vi "getTagDataBytes.vi"(10 "Data Arry":u8[](array[numeric]) format="%x") -> (2 "Bytes":u8)   [LabVIEW 2018]
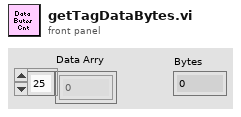
[diagram p1: front panel]
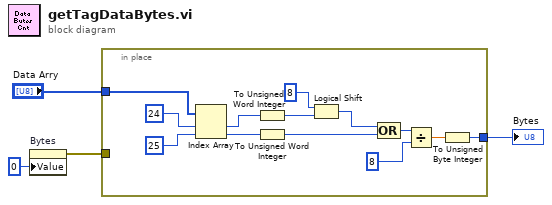
[diagram p0: block diagram]
diagram:
  n1 = property on="Bytes" class="DigNum (strict)"("Value"=u8 0 ("Butes")) -> (error out=w1:errorcluster)  [unwired: 2 in, 1 out]
  n2 = in-place {
    in-place-border: "Data Arry" -> [w17]
    in-place-border: [w5] -> w3
    in-place-border: w1 -> [_]
    n3 = Index Array(array=w17, index #1=24 ("index"), index #2=25 ("index")) -> (element #1=w14:u8, element #2=w13:u8)
    n4 = To Unsigned Word Integer(number=w14) -> (unsigned 16bit integer=w12:u16)
    n5 = To Unsigned Word Integer(number=w13) -> (unsigned 16bit integer=w9:u16)
    n6 = Logical Shift(y=8, x=w12) -> (x << y=w10:u16)
    n7 = Compound Arithmetic op=OR(w10, w9) -> (w8:u16)
    n8 = Divide(x=w8, y=u16 8) -> (x/y=w6:dbl)
    n9 = To Unsigned Byte Integer(number=w6) -> (unsigned 8bit integer=w5:u8)
  }
  "Bytes" <- w3
